vi "Get_Auth_Code.vi"(8 "error in (no error)":errorcluster, 11 "Asana in":refnum<class "Asana.lvclass">) -> (0 "error out":errorcluster, 3 "Asana out":refnum<class "Asana.lvclass">)   [LabVIEW 2016, in "Asana.lvclass"]
uses:
  Asana.lvclass
  Asana.lvclass/Asana.ctl
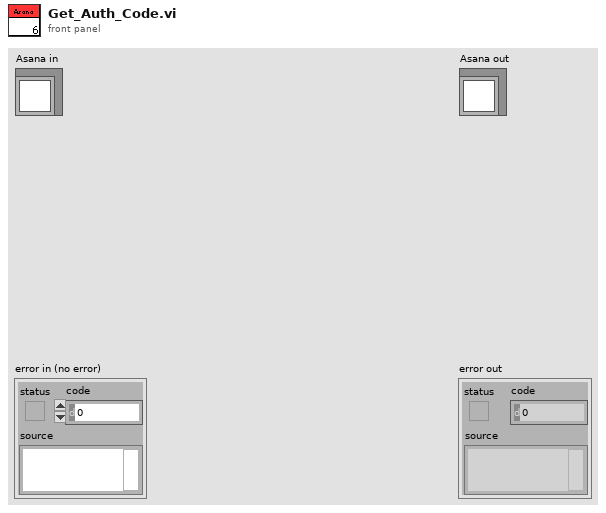
[diagram p1: front panel]
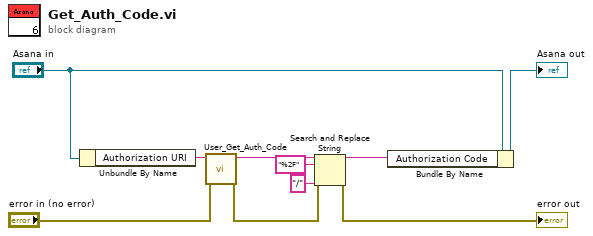
[diagram p0: block diagram]
diagram:
  n1 = Unbundle By Name("Asana in") -> ("Authorization URI"=w8:string)
  n2 = call "User_Get_Auth_Code.vi"("error in (no error)"="error in (no error)", "URL In"=w8) -> ("error out"=w2:errorcluster, "Auth Code"=w4:string)  [unwired: 8 in]
  n3 = Search and Replace String(input string=w4, search string="%2F", replace string="/" ("replace string (\"\")"), error in=w2) -> (result string=w3:string, error out=→"error out":errorcluster)  [unwired: 4 in, 2 out]
  n4 = Bundle By Name(cluster="Asana in", "Authorization Code"=w3) -> (→"Asana out":refnum<class "Asana.lvclass">)
